vi "Find Hardware Type.vi"(0 "Test Results In":T1, 11 "error in (no error)":errorcluster) -> (4 "Test Results Out":T1, 6 "Pass/Fail?":bool, 8 "Report Text":string, 15 "error out":errorcluster)   [LabVIEW 2016]
doc: "This VI searches the config file for the hardware type defined by model number in the Model Config file."
uses:
  controls/Test Results.ctl
  <vilib>/Utility/config.llb/Read Key (String).vi
  <vilib>/Utility/error.llb/Error Cluster From Error Code.vi
  <vilib>/ErrorRing/Error Ring.xnode
  <vilib>/Utility/config.llb/NI_LVConfig.lvlib
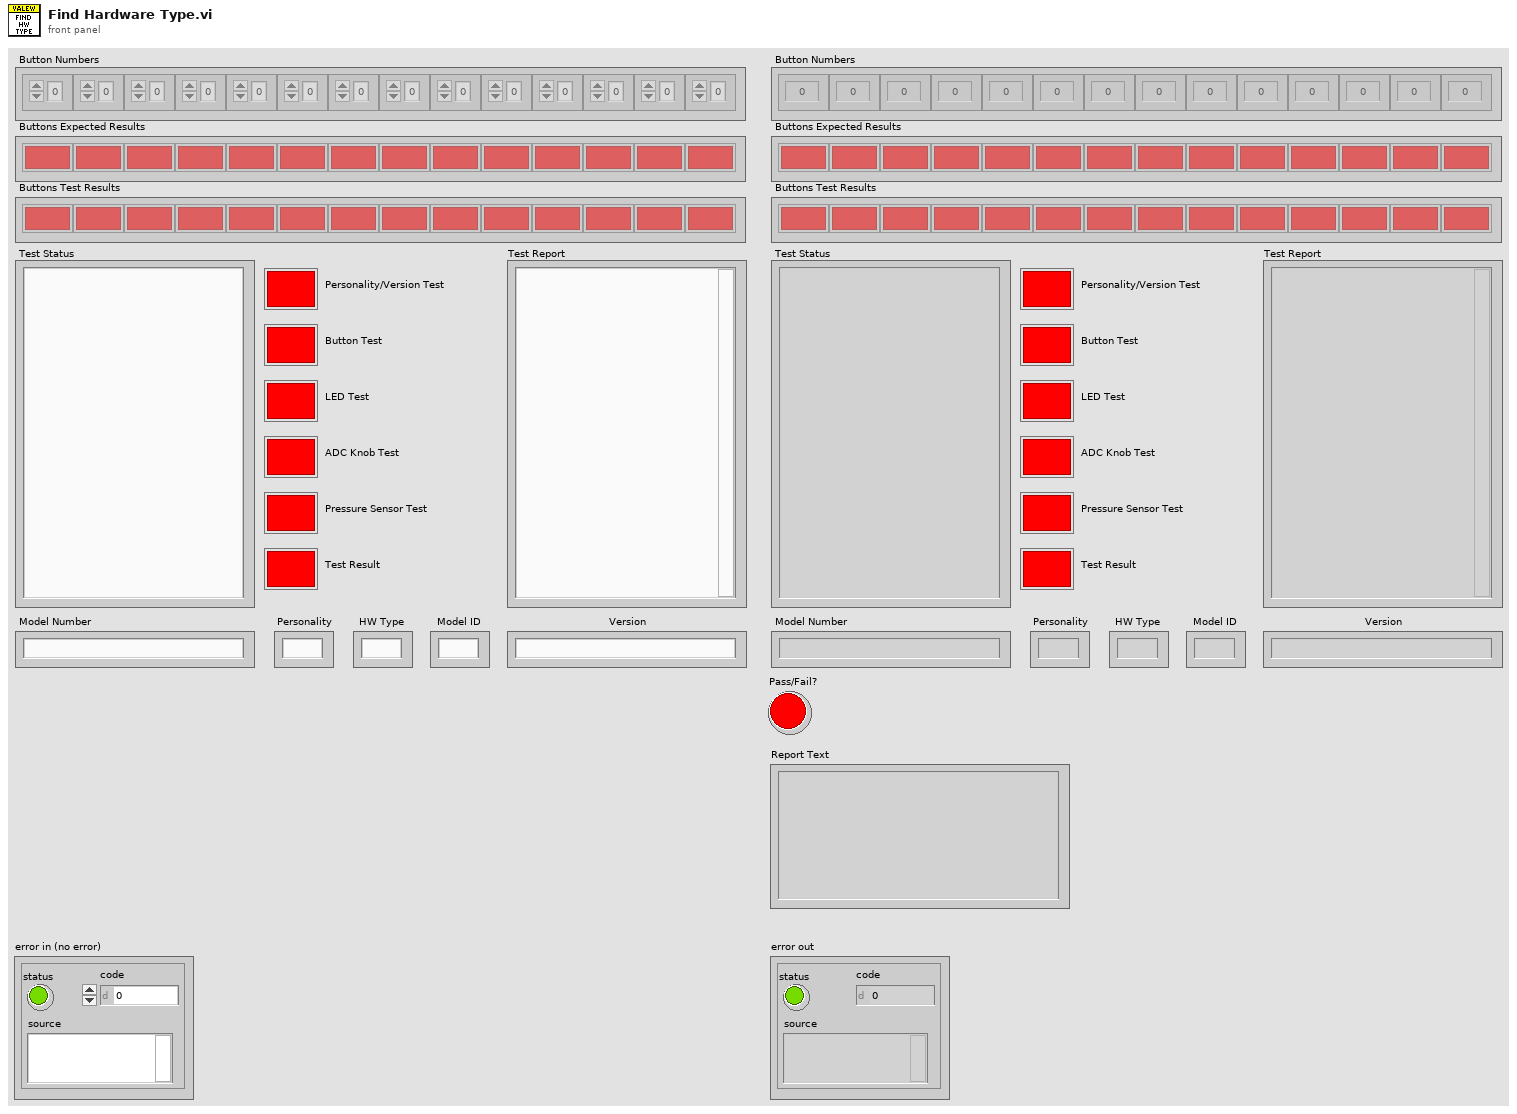
[diagram p1: front panel]
types:
  T1 = typedef "Test Results.ctl" = cluster{"Test Status":string, "Personality/Version Test ":bool, "Test Report":string, "Model Number":string, "Button Numbers":i32[], "Buttons Test Results":bool[], "Buttons Expected Results":bool[], "Model ID":string, "Personality":string, "HW Type":string, "Version":string, "Button Test":bool, "LED Test":bool, "ADC Knob Test":bool, "Pressure Sensor Test":bool, "Test Result":bool}
  T2 = typedef "NI_LVConfig.lvlib/Config Data RefNum.ctl" = refnum<k1>
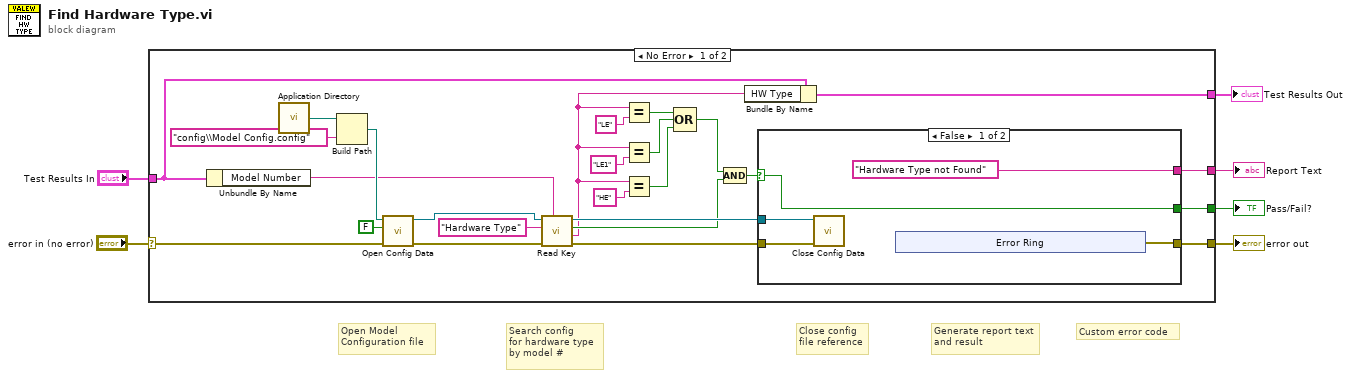
[diagram p0: block diagram]
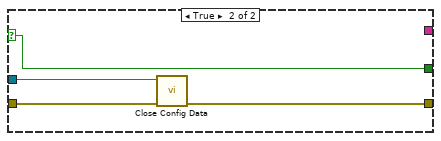
[diagram p2: hidden frame]
diagram:
  # "Custom error code"
  # "Generate report text\nand result"
  # "Close config\nfile reference"
  # "Search config \nfor hardware type\nby model #"
  # "Open Model \nConfiguration file"
  n1 = case shown="No Error" "error in (no error)" {
    selector: "error in (no error)" -> [w22 w47]
    tunnel: [w31 w47] -> w6
    tunnel: [w21 _] -> w4
    tunnel: [w20 _] -> w3
    tunnel: "Test Results In" -> [w18 _]
    tunnel: [w17 _] -> w1
    frame No Error {
      n2 = Unbundle By Name(w18) -> ("Model Number"=w19:string)
      n3 = call <vilib>:"Application Directory.vi"() -> ("Application Directory"=w27:path)
      n4 = Build Path(base path=w27, name or relative path="config\\Model Config.config") -> (appended path=w26:path)
      n5 = call <vilib>:"Open Config Data.vi"("error in (no error)"=w22, "create file if necessary (T)"=FALSE, "configuration file path"=w26) -> ("error out"=w25:errorcluster, "refnum"=w23:T2)  [unwired: 6 in, 1 out]
      n6 = call-poly <vilib>:"Read Key.vi"("section"=w19, "error in (no error)"=w25, "key"="Hardware Type", "refnum"=w23) -> ("error out"=w32:errorcluster, "value"=w8:string, "found?"=w12:bool, "refnum out"=w30:T2)  [unwired: 4 in]
      n7 = Equal?(x=w8, y="LE") -> (x = y?=w14:bool)
      n8 = Equal?(x=w8, y="LE1") -> (x = y?=w13:bool)
      n9 = Equal?(x=w8, y="HE") -> (x = y?=w7:bool)
      n10 = Compound Arithmetic op=OR(w14, w13, w7) -> (w11:bool)
      n11 = Compound Arithmetic op=AND(w11, w12) -> (w10:bool)
      n12 = Bundle By Name(cluster=w18, "HW Type"=w8) -> (w17:T1)
      n13 = case shown="False" w10 {
        selector: w10 -> [w36 w43]
        tunnel: w32 -> [w34 w46]
        tunnel: [w37 w45] -> w31
        tunnel: w30 -> [w33 w44]
        tunnel: [w36 w43] -> w21
        tunnel: ["Hardware Type not Found" _] -> w20
        frame False {
          n14 = call <vilib>:"Close Config Data.vi"("error in (no error)"=w34, "refnum"=w33) -> ()  [unwired: 8 in, 2 out]
          n15 = xnode "Error Ring"() -> ("error out"=w37:errorcluster)
        }
        frame True {
          n16 = call <vilib>:"Close Config Data.vi"("error in (no error)"=w46, "refnum"=w44) -> ("error out"=w45:errorcluster)  [unwired: 8 in, 1 out]
        }
      }
    }
    frame Error {
    }
  }
  "error out" <- w6
  "Report Text" <- w3
  "Pass/Fail?" <- w4
  "Test Results Out" <- w1
